vi "Shooter_HW.vi"() -> ()   [LabVIEW 2017]
uses:
  <vilib>/Rock Robotics/WPI/ThirdParty/CanMotor/TalonSRX/WPI_CANTalonSRX_APIControlMode.ctl
  Globals/Global_STOP.vi
  Global_HoodSensorPosition.vi
  Global_ShooterCTRL.vi
  <vilib>/Rock Robotics/WPI/ThirdParty/CanMotor/TalonSRX/WPI_CANTalonSRX_BrakeOverride.ctl
  <vilib>/Rock Robotics/WPI/ThirdParty/CanMotor/TalonSRX/WPI_CANTalonSRX_APIFeedbackSelect.ctl
  Global_FlyWheelRPM.vi
  TypeDefs/Cluster_SRX PID Values.ctl
  TypeDefs/Cluster_SRX Status With Encoder.ctl
  TypeDefs/Cluster_SRX Limit Switches.ctl
panel:
  out "Hood Limit Switches":T1
  out "RPM Out":dbl format="%#_13g"
  in  "Fly Wheel PID":T2={"P"=0.3, "I"=0.0, "D"=0.0, "F"=0.036, "I Zone"=0.0, "Ramp Rate"=0.0}
  in  "Fly Wheel RPM In":dbl
  in  "T - Vbus\nF - Velocity":bool
  out "Fly Wheel":T3
  out "Hood":T3
  in  "Hood PID":T2={"P"=9.0, "I"=0.0, "D"=8.0, "F"=0.0, "I Zone"=0.0, "Ramp Rate"=0.0}
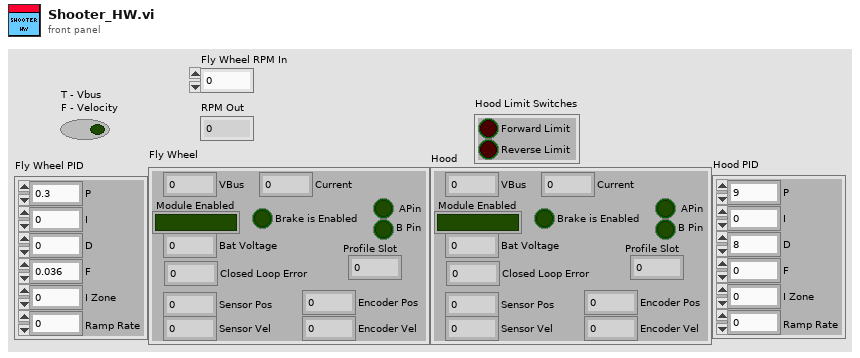
[diagram p1: front panel]
types:
  T1 = typedef "Cluster_SRX Limit Switches.ctl" = cluster{"Forward Limit":bool, "Reverse Limit":bool}
  T2 = typedef "Cluster_SRX PID Values.ctl" = cluster{"P":dbl, "I":dbl, "D":dbl, "F":dbl, "I Zone":dbl, "Ramp Rate":dbl}
  T3 = typedef "Cluster_SRX Status With Encoder.ctl" = cluster{"VBus ":dbl, "Module Enabled":bool, "Closed Loop Error":dbl, "Sensor Pos":dbl, "Sensor Vel":dbl, "Current":dbl, "Brake is Enabled":bool, "Encoder Pos":dbl, "Encoder Vel":dbl, " APin":bool, "B Pin":bool, "Bat Voltage":dbl, "Profile Slot":dbl}
  T4 = typedef "WPI_CANTalonSRX_APIFeedbackSelect.ctl" = enum16{"Digital Quadrature Encoder", "Analog Potentiometer", "Analog Encoder", "Count on Quad-A (Rising-Edge)", "Count on Quad-A (Falling-Edge)", "CTR Magnetic Enc (Absolute)", "CTR Magnetic Enc (Relative)", "Pulse Width"}
  T5 = typedef "WPI_CANTalonSRX_APIControlMode.ctl" = enum8{"Percent VBus", "Speed", "Position", "Slave", "Unchanged / Invalid", "Voltage Compensation", "Current", "Motion Profile", "Motion Magic"}
  T6 = typedef "WPI_CANTalonSRX_BrakeOverride.ctl" = enum8{"No Override", "Override to Coast", "Override to Brake"}
  T7 = typedef "WPI_MotorControlDeviceRef.ctl" = cluster{"DeviceStatus":errorcluster, "Type":T8, "PWM":cluster{"PWM Channel":T9, "DeadBand":T10}, "CAN":cluster{"Device Number":u8, "SetOutput VI Ref":variant, "GetOutput VI Ref":variant, "Enable VI Ref":variant, "Disable VI Ref":variant, "Data":variant}, "Invert":bool}
  T8 = typedef "WPI_MotorControlType.ctl" = enum16{"PWM", "CAN"}
  T9 = typedef "FPGA_DIOPWMChannel.ctl" = enum8{"PWM 0", "PWM 1", "PWM 2", "PWM 3", "PWM 4", "PWM 5", "PWM 6", "PWM 7", "PWM 8", "PWM 9", "PWM MXP 0", "PWM MXP 1", "PWM MXP 2", "PWM MXP 3", "PWM MXP 4", "PWM MXP 5", "PWM MXP 6", "PWM MXP 7", "PWM MXP 8", "PWM MXP 9", "Invalid"}
  T10 = typedef "WPI_PWMDeadband.ctl" = cluster{"Name":string, "maxPositivePwm":i32, "minPositivePwm":i32, "centerPwm":i32, "maxNegativePwm":i32, "minNegativePwm":i32, "angularRange":u16}
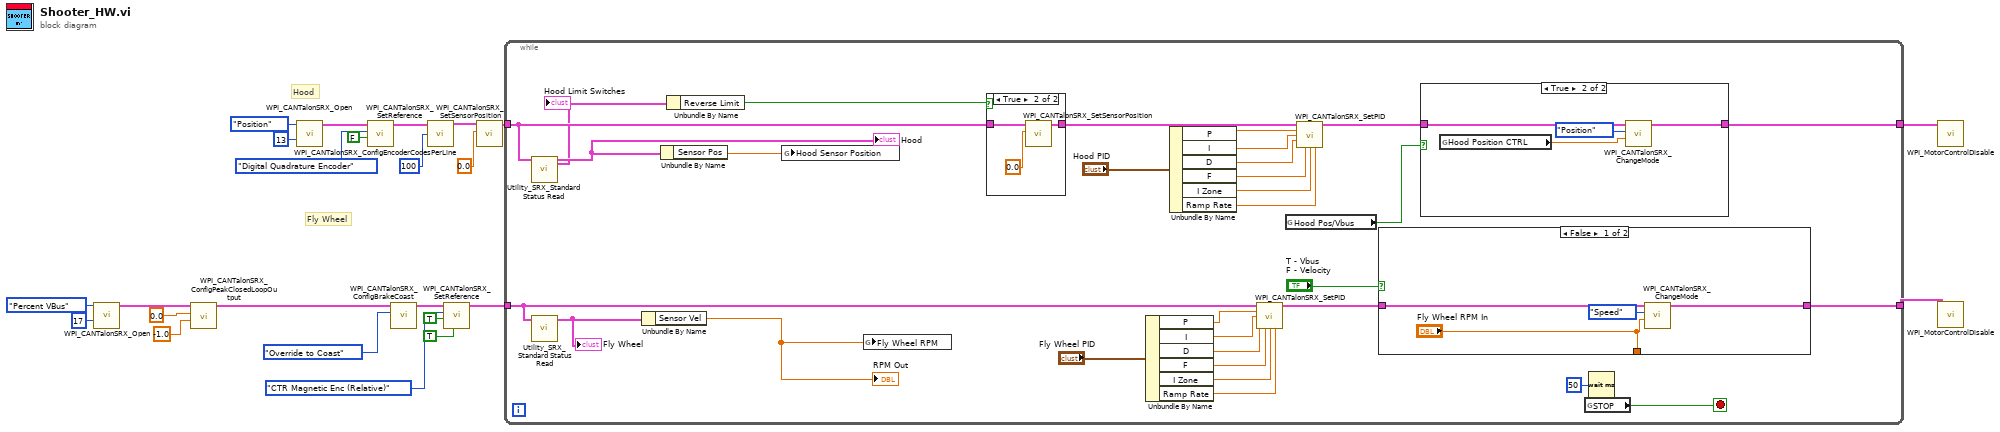
[diagram p0: block diagram]
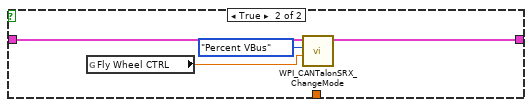
[diagram p2: hidden frame]
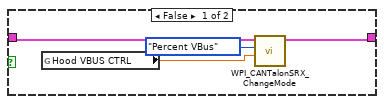
[diagram p4: hidden frame]
diagram:
  # "Fly Wheel"
  # "Hood"
  n1 = call <vilib>:"WPI_CANTalonSRX_Open.vi"("Device Number"=u8 17, "Control Mode"=WPI_CANTalonSRX_APIControlMode."Percent VBus") -> ("CAN Talon SRX Ref"=w5:T7)  [unwired: 8 in, 1 out]
  n2 = call <vilib>:"WPI_CANTalonSRX_ConfigPeakClosedLoopOutput.vi"("Reverse Peak Output"=-1.0, "Forward Peak Output"=0.0, "CAN Talon SRX Ref"=w5) -> ("CAN Talon SRX Ref"=w4:T7)  [unwired: 7 in, 1 out]
  n3 = call <vilib>:"WPI_CANTalonSRX_Open.vi"("Device Number"=u8 13, "Control Mode"=WPI_CANTalonSRX_APIControlMode."Position") -> ("CAN Talon SRX Ref"=w22:T7)  [unwired: 8 in, 1 out]
  n4 = call <vilib>:"WPI_CANTalonSRX_SetReference.vi"("Reverse Feedback Sensor"=FALSE, "Feedback Reference"=WPI_CANTalonSRX_APIFeedbackSelect."Digital Quadrature Encoder", "CAN Talon SRX Ref"=w22) -> ("CAN Talon SRX Ref"=w21:T7)  [unwired: 7 in, 1 out]
  n5 = call <vilib>:"WPI_CANTalonSRX_ConfigBrakeCoast.vi"("Brake / Coast Mode"=WPI_CANTalonSRX_BrakeOverride."Override to Coast", "CAN Talon SRX Ref"=w4) -> ("CAN Talon SRX Ref"=w9:T7)  [unwired: 8 in, 1 out]
  n6 = call <vilib>:"WPI_CANTalonSRX_ConfigEncoderCodesPerLine.vi"("CAN Talon SRX Ref"=w21, "Number Encoder Lines\n(Counts Per Rotation)"=u32 100 ("Number Encoder Lines\n(Counts Per Rotation)")) -> ("CAN Talon SRX Ref"=w10:T7)  [unwired: 12 in, 1 out]
  n7 = call <vilib>:"WPI_CANTalonSRX_SetReference.vi"("Reverse Closed-Loop Output"=TRUE, "Reverse Feedback Sensor"=TRUE, "Feedback Reference"=WPI_CANTalonSRX_APIFeedbackSelect."CTR Magnetic Enc (Relative)", "CAN Talon SRX Ref"=w9) -> ("CAN Talon SRX Ref"=w8:T7)  [unwired: 6 in, 1 out]
  n8 = call <vilib>:"WPI_CANTalonSRX_SetSensorPosition.vi"("New Sensor Position"=0.0, "CAN Talon SRX Ref"=w10) -> ("CAN Talon SRX Ref"=w11:T7)  [unwired: 8 in, 1 out]
  n9 = while {
    tunnel: [w41] -> w24
    tunnel: [w54] -> w23
    tunnel: w8 -> [w29]
    tunnel: w11 -> [w31]
    stop <- w55 stop-if-true
    n10 = call "Utility_SRX_Standard Status Read.vi"("SingleMotorRef"=w31) -> ("SRX With Encoder Out"=w28:T3, "SRX Limit Swiths Out"=w25:T1)  [unwired: 8 in, 1 out]
    "Hood" <- w28
    "Hood Limit Switches" <- w25
    n11 = call "Utility_SRX_Standard Status Read.vi"("SingleMotorRef"=w29) -> ("SRX With Encoder Out"=w27:T3)  [unwired: 8 in, 2 out]
    "Fly Wheel" <- w27
    n12 = Unbundle By Name(w27) -> ("Sensor Vel"=w26:dbl)
    "RPM Out" <- w26
    n13 = Unbundle By Name(w28) -> ("Sensor Pos"=w42:dbl)
    n14 = Unbundle By Name(w25) -> ("Reverse Limit"=w30:bool)
    n15 = global write "Global_HoodSensorPosition.vi" "Hood Sensor Position"(w42) -> ()
    n16 = global write "Global_FlyWheelRPM.vi" "Fly Wheel RPM"(w26) -> ()
    n17 = case shown="True" w30 {
      tunnel: [w64 w66] -> w43
      tunnel: w31 -> [w64 w65]
      frame False {
      }
      frame True {
        n18 = call <vilib>:"WPI_CANTalonSRX_SetSensorPosition.vi"("New Sensor Position"=0.0, "CAN Talon SRX Ref"=w65) -> ("CAN Talon SRX Ref"=w66:T7)  [unwired: 8 in, 1 out]
      }
    }
    n19 = Unbundle By Name("Fly Wheel PID") -> ("P"=w38:dbl, "I"=w37:dbl, "D"=w36:dbl, "F"=w35:dbl, "I Zone"=w34:dbl, "Ramp Rate"=w33:dbl)
    n20 = Unbundle By Name("Hood PID") -> ("P"=w47:dbl, "I"=w48:dbl, "D"=w46:dbl, "F"=w49:dbl, "I Zone"=w51:dbl, "Ramp Rate"=w50:dbl)
    n21 = call <vilib>:"WPI_CANTalonSRX_SetPID.vi"("CAN Talon SRX Ref"=w29, "P"=w38, "I"=w37, "D"=w36, "F"=w35, "I Zone"=w34, "Ramp Rate"=w33) -> ("CAN Talon SRX Ref"=w32:T7)  [unwired: 7 in, 1 out]
    n22 = global read "Global_ShooterCTRL.vi" "Hood Pos/Vbus"() -> (w44:bool)
    n23 = call <vilib>:"WPI_CANTalonSRX_SetPID.vi"("CAN Talon SRX Ref"=w43, "P"=w47, "I"=w48, "D"=w46, "F"=w49, "I Zone"=w51, "Ramp Rate"=w50) -> ("CAN Talon SRX Ref"=w45:T7)  [unwired: 7 in, 1 out]
    n24 = case shown="False" "T - Vbus\nF - Velocity" {
      tunnel: [w58 w63] -> w54
      tunnel: w32 -> [w57 w60]
      tunnel: ["Fly Wheel RPM In" _] -> _
      frame False {
        n25 = call <vilib>:"WPI_CANTalonSRX_ChangeMode.vi"("Output"="Fly Wheel RPM In", "Control Mode"=WPI_CANTalonSRX_APIControlMode."Speed", "CAN Talon SRX Ref"=w57) -> ("CAN Talon SRX Ref"=w58:T7)  [unwired: 7 in, 1 out]
      }
      frame True {
        n26 = global read "Global_ShooterCTRL.vi" "Fly Wheel CTRL"() -> (w61:dbl)
        n27 = call <vilib>:"WPI_CANTalonSRX_ChangeMode.vi"("Output"=w61, "Control Mode"=WPI_CANTalonSRX_APIControlMode."Percent VBus", "CAN Talon SRX Ref"=w60) -> ("CAN Talon SRX Ref"=w63:T7)  [unwired: 7 in, 1 out]
      }
    }
    n28 = case shown="True" w44 {
      tunnel: w45 -> [w68 w75]
      tunnel: [w69 w72] -> w41
      frame False {
        n29 = global read "Global_ShooterCTRL.vi" "Hood VBUS CTRL"() -> (w70:dbl)
        n30 = call <vilib>:"WPI_CANTalonSRX_ChangeMode.vi"("Output"=w70, "Control Mode"=WPI_CANTalonSRX_APIControlMode."Percent VBus", "CAN Talon SRX Ref"=w68) -> ("CAN Talon SRX Ref"=w69:T7)  [unwired: 7 in, 1 out]
      }
      frame True {
        n31 = global read "Global_ShooterCTRL.vi" "Hood Position CTRL"() -> (w73:dbl)
        n32 = call <vilib>:"WPI_CANTalonSRX_ChangeMode.vi"("Output"=w73, "Control Mode"=WPI_CANTalonSRX_APIControlMode."Position", "CAN Talon SRX Ref"=w75) -> ("CAN Talon SRX Ref"=w72:T7)  [unwired: 7 in, 1 out]
      }
    }
    n33 = global read "Global_Stop.vi" "STOP"() -> (w55:bool)
    n34 = Wait (ms)(milliseconds to wait=u32 50) -> ()  [unwired: 1 out]
  }
  n35 = call <vilib>:"WPI_MotorControlDisable.vi"("MotorControlDevRef"=w24) -> ()  [unwired: 9 in, 2 out]
  n36 = call <vilib>:"WPI_MotorControlDisable.vi"("MotorControlDevRef"=w23) -> ()  [unwired: 9 in, 2 out]
